vi "CODCr质控流程 (子VI).vi"(10 "CODCr量程切换":enum32{"H", "L", "AUTO"}(ring)=enum."AUTO", 11 "COD":bool) -> (2 "CODCr中断报警":bool, 3 "布尔":bool)   [LabVIEW 2016, in "质控单元.lvlib"]
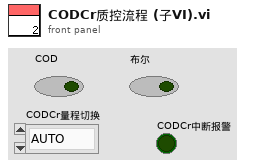
[diagram p1: front panel]
types:
  T1 = enum16{"待机", "启动水样测量", "水样测量中", "启动加标", "启动加标回收", "加标回收测量中", "结束"}
  T2 = cluster{"测量模式":enum16{"水样测量", "标样核查", "零点核查", "跨度核查", "空白测试", "加标回收", "平行样", "校零", "校标"}}
  T3 = enum16{"空闲", "水样测试", "标样核查", "零点核查", "跨度核查", "空白测试", "平行样测试", "加标回收", "空白校准", "标样校准", "初始化（清洗）"}
  T4 = cluster{"因子编码":u32, "单位":u16, "标样参考值":sgl, "水样数据时间":timestamp, "水样实测值":sgl, "水样数据标识":string, "标样数据时间":timestamp, "标样实测值":sgl, "标样数据标识":string, "空白数据时间":timestamp, "空白实测值":sgl, "空白数据标识":string, "零点核查数据时间":timestamp, "零点核查实测值":sgl, "零点核查数据标识":string, "跨度核查数据时间":timestamp, "跨度核查实测值":sgl, "跨度核查数据标识":string, "加标回收数据时间":timestamp, "加标回收实测值":sgl, "加标回收数据标识":string, "平行样数据时间":timestamp, "平行样实测值":sgl, "平行样数据标识":string}
  T5 = cluster{"量程":dbl, "检出限":dbl, "加标前水样浓度":dbl, "加标后水样浓度":dbl, "加标水杯定容体积":dbl, "加标母液浓度":dbl, "加标体积":dbl, "加标回收率":dbl}
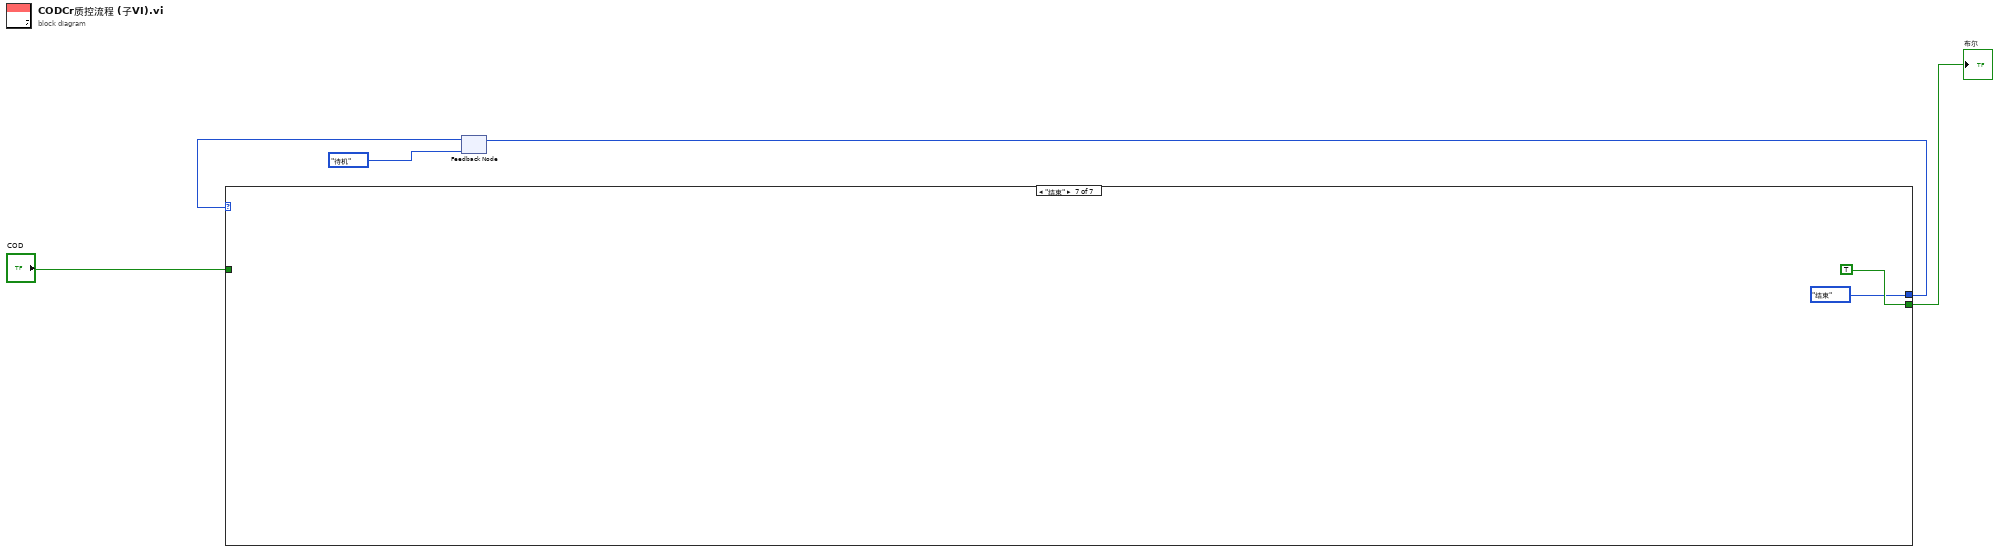
[diagram p0: block diagram]
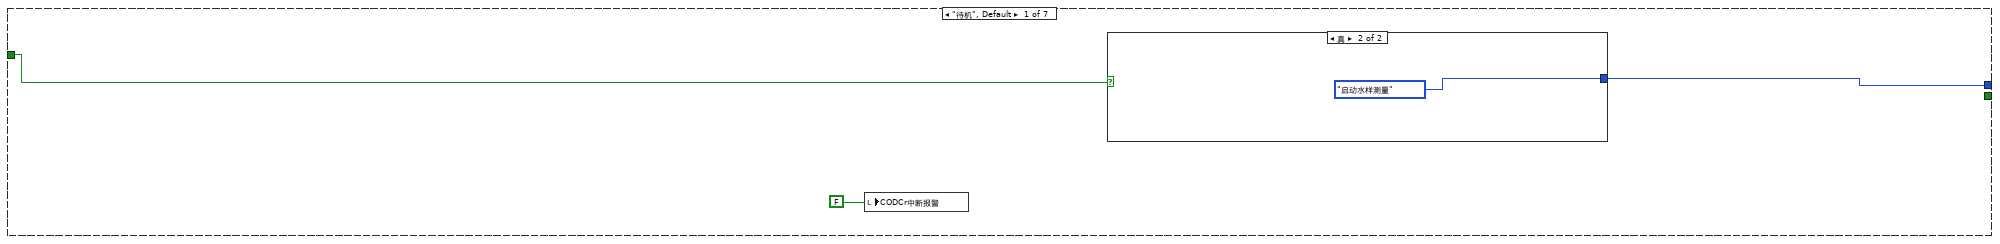
[diagram p2: hidden frame]
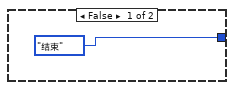
[diagram p3: hidden frame]
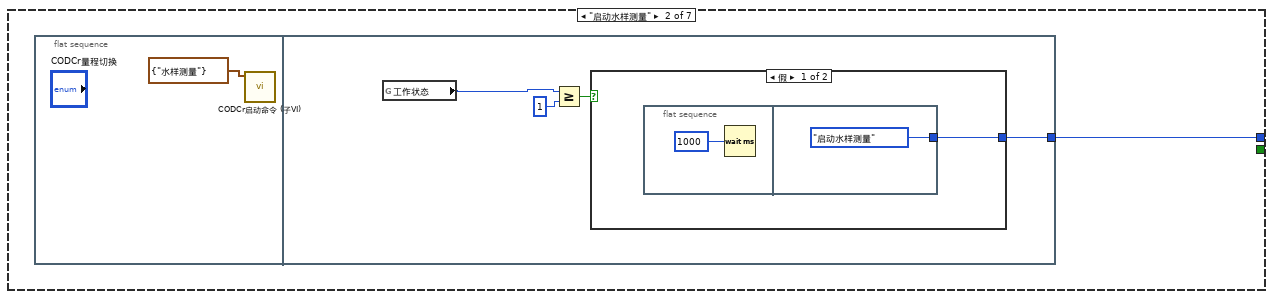
[diagram p4: hidden frame]
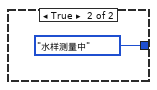
[diagram p5: hidden frame]
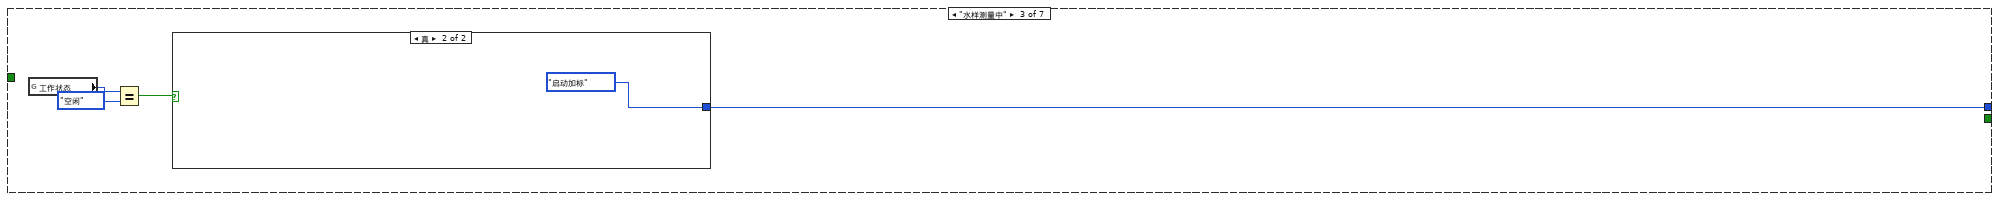
[diagram p6: hidden frame]
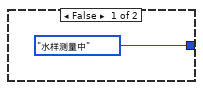
[diagram p7: hidden frame]
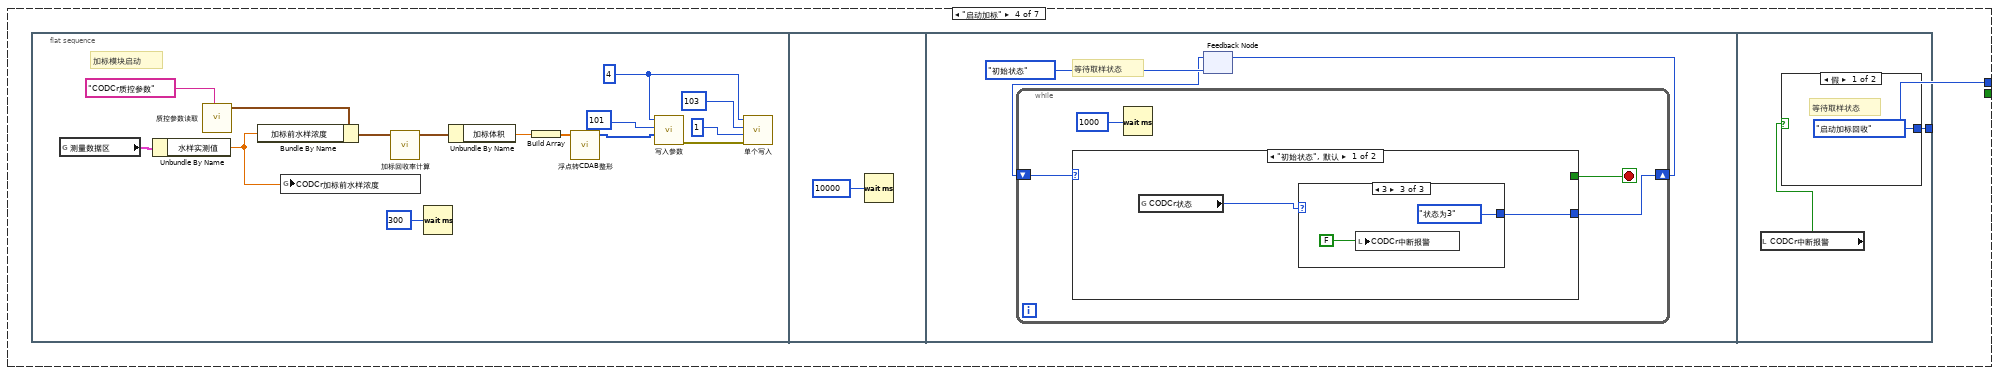
[diagram p8: hidden frame]
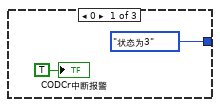
[diagram p9: hidden frame]
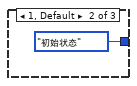
[diagram p10: hidden frame]
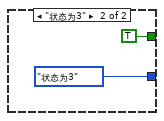
[diagram p11: hidden frame]
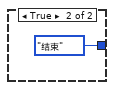
[diagram p12: hidden frame]
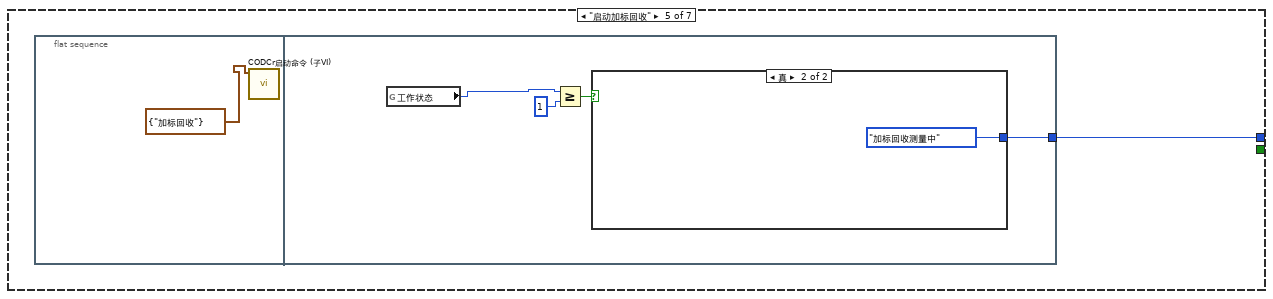
[diagram p13: hidden frame]
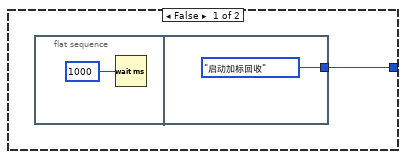
[diagram p14: hidden frame]
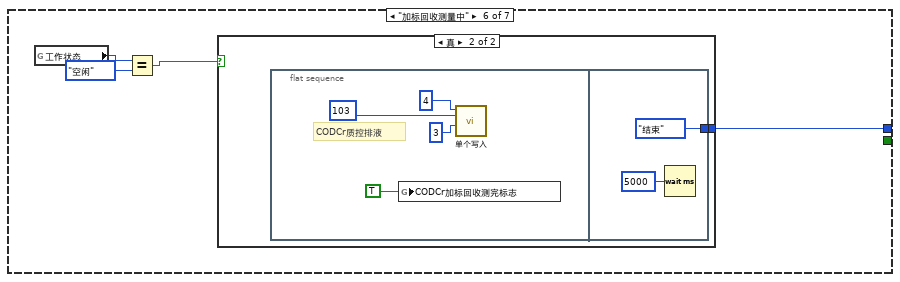
[diagram p15: hidden frame]
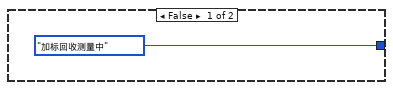
[diagram p16: hidden frame]
diagram:
  n1 = feedback #1(T1."待机") -> (w3:T1)
  n2 = case shown="\"结束\"" w3 {
    tunnel: [w8 w11 w24 w27 w64 w77 T1."结束"] -> w4
    tunnel: [_ _ _ _ _ _ TRUE] -> w2
    tunnel: "COD" -> [w7 _ _ _ _ _ _]
    frame "待机", Default {
      n3 = local write "CODCr中断报警"(FALSE ("CODMn中断报警")) -> ()
      n4 = case shown="真" w7 {
        tunnel: [T1."结束" T1."启动水样测量"] -> w8
        frame False {
        }
        frame True {
        }
      }
    }
    frame "启动水样测量" {
      n5 = flat-sequence {
        tunnel: [w14] -> w11
        frame #0 {
          n6 = call "CODCr启动命令 (子VI).vi"("启动测量模式"=T2 {"测量模式"=enum."水样测量"}) -> ()  [unwired: 11 in]
        }
        frame #1 {
          n7 = global read "CODcr全局变量.vi" "工作状态"() -> (w13:T3)
          n8 = Greater Or Equal?(x=w13, y=1) -> (x >= y?=w16:bool)
          n9 = case shown="假" w16 {
            tunnel: [w17 T1."水样测量中"] -> w14
            frame False {
              n10 = flat-sequence {
                tunnel: [T1."启动水样测量"] -> w17
                frame #0 {
                  n11 = Wait (ms)(milliseconds to wait=u32 1000 ("等待时间（毫秒）")) -> ()  [unwired: 1 out]
                }
                frame #1 {
                }
              }
            }
            frame True {
            }
          }
        }
      }
    }
    frame "水样测量中" {
      n12 = global read "CODcr全局变量.vi" "工作状态"() -> (w23:T3)
      n13 = Equal?(x=w23, y=T3."空闲") -> (x = y?=w21:bool)
      n14 = case shown="真" w21 {
        tunnel: [T1."水样测量中" T1."启动加标"] -> w24
        frame False {
        }
        frame True {
        }
      }
    }
    frame "启动加标" {
      n15 = flat-sequence {
        tunnel: [w61] -> w27
        frame #0 {
          w31 = u16 4 ("value")
          # "加标模块启动"
          n16 = global read "CODcr全局变量.vi" "测量数据区"() -> (w29:T4)
          n17 = Unbundle By Name(w29) -> ("水样实测值"=w28:sgl)
          n18 = call "质控参数读取.vi"("section"="CODCr质控参数") -> ("参数"=w40:T5)  [unwired: 9 in, 1 out]
          n19 = Bundle By Name(cluster=w40, "加标前水样浓度"=w28) -> (w41:T5)
          n20 = global write "水样浓度全局.vi" "CODCr加标前水样浓度"(w28) -> ()
          n21 = call "加标回收率计算.vi"("参数"=w41) -> ("参数 out"=w39:T5)  [unwired: 10 in]
          n22 = Wait (ms)(milliseconds to wait=u32 300 ("等待时间（毫秒）")) -> ()  [unwired: 1 out]
          n23 = Unbundle By Name(w39) -> ("加标体积"=w32:dbl)
          n24 = Build Array(w32) -> (w38:dbl[])
          n25 = call "浮点转CDAB整形.vi"("浮点数"=w38) -> ("CDAB整形输出"=w33:u16[])  [unwired: 10 in]
          n26 = call "写入参数.vi"("values"=w33, "starting address"=u16 101, "Slave ID"=w31) -> ("error out"=w37:errorcluster)  [unwired: 8 in]
          n27 = call "单个写入.vi"("Error in"=w37, "value"=u16 1, "address"=u16 103, "Slave ID"=w31) -> ()  [unwired: 7 in, 1 out]
        }
        frame #1 {
          n28 = Wait (ms)(milliseconds to wait=u32 10000 ("等待时间（毫秒）")) -> ()  [unwired: 1 out]
        }
        frame #2 {
          # "等待取样状态"
          n29 = feedback #2(enum16{"初始状态", "状态为3"}."初始状态") -> (w45:enum16{"初始状态", "状态为3"})
          n30 = while {
            shift-right: [w49] -> w44
            shift-left: w45 -> [w50]
            stop <- w48 stop-if-true
            n31 = case shown="\"初始状态\", 默认" w50 {
              tunnel: [w52 enum16{"初始状态", "状态为3"}."状态为3"] -> w49
              tunnel: [_ TRUE] -> w48
              frame "初始状态", Default {
                n32 = global read "氨氮加标回收状态全局变量.vi" "CODCr状态"() -> (w51:u16)
                n33 = case shown="3" w51 {
                  tunnel: [enum16{"初始状态", "状态为3"}."状态为3" enum16{"初始状态", "状态为3"}."初始状态" enum16{"初始状态", "状态为3"}."状态为3"] -> w52
                  frame 0 {
                    "CODCr中断报警" <- TRUE ("CODMn中断报警")
                  }
                  frame 1, Default {
                  }
                  frame 3 {
                    n34 = local write "CODCr中断报警"(FALSE ("CODMn中断报警")) -> ()
                  }
                }
              }
              frame "状态为3" {
              }
            }
            n35 = Wait (ms)(milliseconds to wait=u32 1000 ("等待时间（毫秒）")) -> ()  [unwired: 1 out]
          }
          n36 = feedback-in #2(w44) -> ()
        }
        frame #3 {
          n37 = local read "CODCr中断报警"() -> (w60:bool)
          n38 = case shown="假" w60 {
            tunnel: [T1."启动加标回收" T1."结束"] -> w61
            frame False {
              # "等待取样状态"
            }
            frame True {
            }
          }
        }
      }
    }
    frame "启动加标回收" {
      n39 = flat-sequence {
        tunnel: [w67] -> w64
        frame #0 {
          n40 = call "CODCr启动命令 (子VI).vi"("启动测量模式"=T2 {"测量模式"=enum."加标回收"}) -> ()  [unwired: 11 in]
        }
        frame #1 {
          n41 = global read "CODcr全局变量.vi" "工作状态"() -> (w66:T3)
          n42 = Greater Or Equal?(x=w66, y=1) -> (x >= y?=w68:bool)
          n43 = case shown="真" w68 {
            tunnel: [w70 T1."加标回收测量中"] -> w67
            frame False {
              n44 = flat-sequence {
                tunnel: [T1."启动加标回收"] -> w70
                frame #0 {
                  n45 = Wait (ms)(milliseconds to wait=u32 1000 ("等待时间（毫秒）")) -> ()  [unwired: 1 out]
                }
                frame #1 {
                }
              }
            }
            frame True {
            }
          }
        }
      }
    }
    frame "加标回收测量中" {
      n46 = global read "CODcr全局变量.vi" "工作状态"() -> (w76:T3)
      n47 = Equal?(x=w76, y=T3."空闲") -> (x = y?=w74:bool)
      n48 = case shown="真" w74 {
        tunnel: [T1."加标回收测量中" w79] -> w77
        frame False {
        }
        frame True {
          n49 = flat-sequence {
            tunnel: [T1."结束"] -> w79
            frame #0 {
              # "CODCr质控排液"
              n50 = global write "质控测完标志全局 1.vi" "CODCr加标回收测完标志"(TRUE ("COD加标回收测完标志")) -> ()
              n51 = call "单个写入.vi"("value"=u16 3, "address"=u16 103, "Slave ID"=u8 4) -> ()  [unwired: 8 in, 1 out]
            }
            frame #1 {
              n52 = Wait (ms)(milliseconds to wait=u32 5000 ("等待时间（毫秒）")) -> ()  [unwired: 1 out]
            }
          }
        }
      }
    }
    frame "结束" {
    }
  }
  "布尔" <- w2
  n53 = feedback-in #1(w4) -> ()
